vi "Add Noise SubVI.vi"(1 "Input 3":u8[][](array[numeric]), 4 "Noise Amplitude":dbl=1.0000000000000002 format="%0.2f", 5 "Choose Noise":string(combo), 6 "seed":i32=-1, 7 "Input 1":u8[][](array[numeric]), 8 "Input 2":u8[][](array[numeric]), 9 "right":i16, 10 "bottom":i16, 11 "deviation":dbl=1.0000000000000002 format="%0.2f") -> (0 "Output 3":u8[][](array[numeric]), 2 "Output 2":u8[][](array[numeric]), 3 "Output 1":u8[][](array[numeric]))   [LabVIEW 2016]
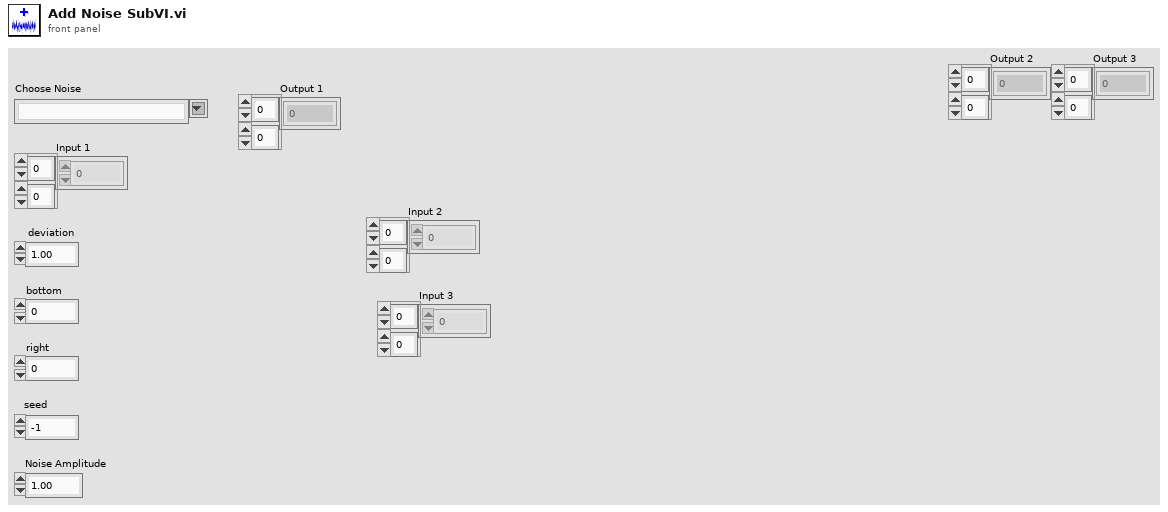
[diagram p1: front panel]
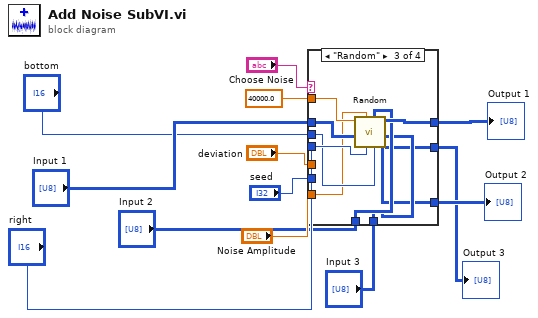
[diagram p0: block diagram]
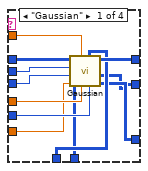
[diagram p2: hidden frame]
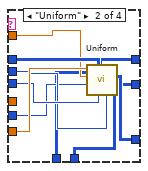
[diagram p3: hidden frame]
diagram:
  n1 = case shown="\"Random\"" "Choose Noise" {
    tunnel: "Input 1" -> [w25 w32 w45 w49]
    tunnel: "deviation" -> [w24 _ _ _]
    tunnel: "seed" -> [w23 w33 _ _]
    tunnel: [w22 w31 w46 w49] -> w7
    tunnel: "bottom" -> [w21 w34 w42 _]
    tunnel: "right" -> [w20 w35 w43 _]
    tunnel: "Noise Amplitude" -> [w19 w36 w37 _]
    tunnel: 40000.0 ("samples") -> [w18 w30 w44 _]
    tunnel: "Input 2" -> [w17 w29 w41 w48]
    tunnel: "Input 3" -> [w16 w28 w40 w47]
    tunnel: [w15 w27 w39 w48] -> w2
    tunnel: [w14 w26 w38 w47] -> w1
    frame "Gaussian" {
      n2 = call "Gaussian.vi"("Intput 3"=w16, "seed"=w23, "Input 2"=w17, "standard deviation"=w24, "samples"=w18, "Amplify"=w19, "right"=w20, "bottom"=w21, "Input 1"=w25) -> ("Output 3"=w15:u8[][], "Output 2"=w14:u8[][], "Output 1"=w22:u8[][])
    }
    frame "Uniform" {
      n3 = call "Uniform.vi"("Input 3"=w28, "bottom"=w34, "Input 2"=w29, "right"=w35, "Input 1"=w32, "seed in"=w33, "samples"=w30, "Numeric"=w36) -> ("Output 3"=w26:u8[][], "Output 2"=w27:u8[][], "Output 1"=w31:u8[][])  [unwired: 1 in]
    }
    frame "Random" {
      n4 = call "Random.vi"("Input 3"=w40, "dimension size 2"=w42, "Input 2"=w41, "dimension size"=w43, "seed"=w37, "Input 1"=w45, "Numeric"=w44) -> ("Output 3"=w38:u8[][], "Output 2"=w39:u8[][], "Output 1"=w46:u8[][])  [unwired: 2 in]
    }
    frame "No noise", Default {
    }
  }
  "Output 1" <- w7
  "Output 2" <- w2
  "Output 3" <- w1
